vi "ProstateParams.vi"(6 "Divide By":u32, 7 "Attenuation":u8(slide) scale=0.0..63.0, 8 "frames":i32=1, 9 "File Name":string, 10 "Patient Info":T1={"ID"="test", "Extended ID"="", "age"=0, "gender"="", "previously\nscanned"="N", "PSA"=0.0, "LOS"=1, "Ethnicty"=3, "Race"=3} {"Race" items=["Am Ind or Alaska", "Asian", "Hawaiian, Pac Isl", "Black or Afr Amer", "White", "more than one race", "unknown"]; "Ethnicty" items=["Hispanic", "Non-Hispanic", "unknown"]; "LOS" items=["1", "2", "3", "4", "5"]; "PSA" format="%.1f"}, 11 "Gage Params":T2={"Capture Config"={"Capture Mode"=0, "Sample Rate"=0, "Multiple Record"=0, "MulRec Acqs"=0}, "Input Config"={"Ch A Coupling"=0, "Ch A Input Range"=0, "Ch B Coupling"=0, "Ch B Input Range"=0}, "Trigger Config"={"Source"=0, "Slope"=0, "Coupling"=0, "Trig Input Range"=0, "Level (mV)"=0, "Trig Depth"=0}, "Transferred"={"Start Point"=0, "Number of Points"=1024, "Mulrec Group"=0}, "Vector Trigger Line"=3, "Total Delay (ms)"=0.0} {"Total Delay (ms)" format="%.2f"; "Vector Trigger Line" min=2 max=315; "Transferred"."Number of Points" min=0 max=8388608; "Transferred"."Start Point" min=-8388608 max=8388608}) -> (3 "Scan Params":T3 {"Att dB" format="%.2f"; "dig dB" format="%.2f"; "Total Delay (ms)" format="%.2f"; "Vert Gain" format="%.2f"})   [LabVIEW 2022 SP3]
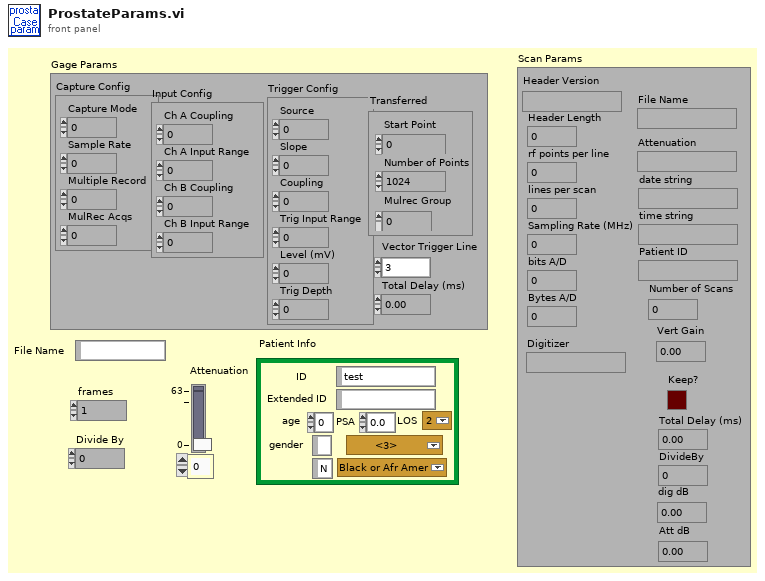
[diagram p1: front panel]
types:
  T1 = cluster{"ID":string, "Extended ID":string, "age":u16, "gender":string, "previously\nscanned":string, "PSA":sgl, "LOS":u8, "Ethnicty":u8, "Race":u8}
  T2 = cluster{"Capture Config":cluster{"Capture Mode":i16, "Sample Rate":i32, "Multiple Record":i16, "MulRec Acqs":i16}, "Input Config":cluster{"Ch A Coupling":i16, "Ch A Input Range":i16, "Ch B Coupling":i16, "Ch B Input Range":i16}, "Trigger Config":cluster{"Source":u16, "Slope":u16, "Coupling":u16, "Trig Input Range":i16, "Level (mV)":i16, "Trig Depth":i32}, "Transferred":cluster{"Start Point":i32, "Number of Points":i32, "Mulrec Group":i32}, "Vector Trigger Line":i16, "Total Delay (ms)":sgl}
  T3 = cluster{"Header Version":string, "Header Length":i32, "rf points per line":u16, "lines per scan":u16, "Sampling Rate (MHz)":i32, "bits A/D":i32, "Bytes A/D":i32, "Digitizer":string, "File Name":string, "Attenuation":string, "date string":string, "time string":string, "Patient ID":string, "Number of Scans":i32, "Vert Gain":dbl, "Keep?":bool, "Total Delay (ms)":sgl, "DivideBy":u32, "dig dB":sgl, "Att dB":sgl}
  T4 = cluster{string, i32, "Number of Points":i32, dbl, dbl, "bits A/D":i32, "Bytes A/D":i32, "Digitizer":string, string, string, "date string":string, "time string":string, "ID":string, "frames":i32, "Scaling Factor":dbl, "Save?":bool, "Total Delay (ms)":sgl, "Divide By":u32, i32, "Attenuation":u8}
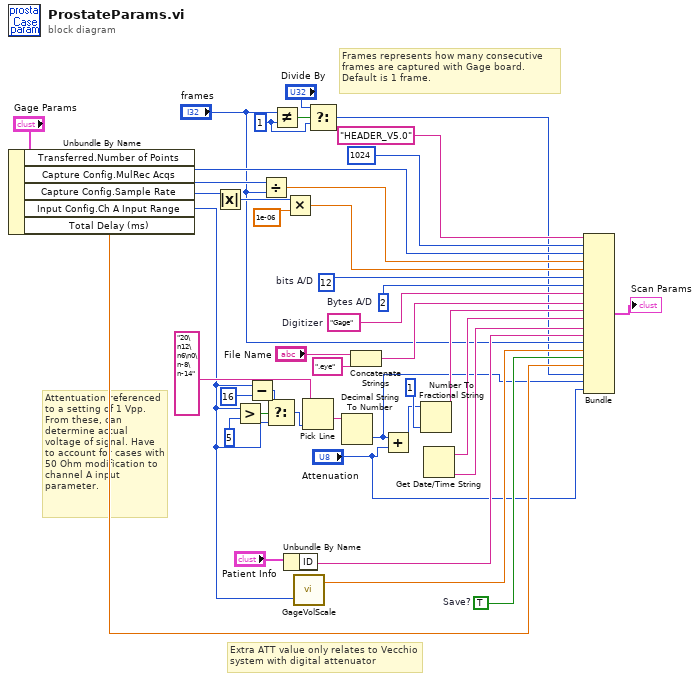
[diagram p0: block diagram]
diagram:
  w4 = 1
  w30 = TRUE  # Save?
  w40 = 12  # bits A/D
  w41 = 2  # Bytes A/D
  w42 = "Gage"  # Digitizer
  # "Extra ATT value only relates to Vecchio system with digital attenuator"
  # "Frames represents how many consecutive frames are captured with Gage board. Default is 1 frame."
  # "Attentuation referenced\nto a setting of 1 Vpp. From these, can determine actual voltage of signal. Have to account for cases with 50 Ohm modification to channel A input parameter."
  n1 = Unbundle By Name("Gage Params") -> ("Transferred.Number of Points"=w29:i32, "Capture Config.MulRec Acqs"=w13:i16, "Capture Config.Sample Rate"=w28:i32, "Input Config.Ch A Input Range"=w9:i16, "Total Delay (ms)"=w11:sgl)
  n2 = Absolute Value(x=w28) -> (abs(x)=w10:i32)
  n3 = Greater?(x=w9, y=5) -> (0:w18:bool)
  n4 = Subtract(x=w9, y=16) -> (x-y=w16:i32)
  n5 = Divide(x=w13, y="frames") -> (x/y=w12:dbl)
  n6 = Select(t=w16, s=w18, f=w9) -> (s? t:f=w15:i32)
  n7 = Not Equal?(x="frames", y=w4) -> (x != y?=w6:bool)
  n8 = Unbundle By Name("Patient Info") -> ("ID"=w21:string)
  n9 = Multiply(x=w10, y=1e-06) -> (x*y=w27:dbl)
  n10 = call "GageVolScale.vi"("Voltage Scale"=w9) -> ("Scaling Factor"=w24:dbl)  [unwired: 2 out]
  n11 = Pick Line(multi-line string="20\n12\n6\n0\n-8\n-14", line index=w15) -> (output string=w31:string)  [unwired: 1 out]
  n12 = Select(t="Divide By", s=w6, f=w4) -> (s? t:f=w5:u32)
  n13 = Decimal String To Number(string=w31) -> (number=w2:i32)  [unwired: 3 out]
  n14 = Concatenate Strings("File Name", ".eye") -> (w34:string)
  n15 = Add(x=w2, y="Attenuation") -> (x+y=w8:i32)
  n16 = Number To Fractional String(number=w8, precision (6)=i16 1) -> (F-format string=w35:string)  [unwired: 2 out]
  n17 = Get Date/Time String() -> (date string=w33:string, time string=w32:string)  [unwired: 3 out]
  n18 = Bundle("HEADER_V5.0", 1024, "Number of Points"=w29, w12, w27, "bits A/D"=w40, "Bytes A/D"=w41, "Digitizer"=w42, w34, w35, "date string"=w33, "time string"=w32, "ID"=w21, "frames"="frames", "Scaling Factor"=w24, "Save?"=w30, "Total Delay (ms)"=w11, "Divide By"=w5, w2, "Attenuation"="Attenuation") -> (→"Scan Params":T4)  [unwired: 1 out]
